vi "Drop Message Core.vi"(11 "Process Job Msg in":refnum<class "Process Job Msg.lvclass">) -> ()   [LabVIEW 2023, in "Worker.lvlib" / "Process Job Msg.lvclass"]
doc: "(<B>Filename</B>: Actor Framework.lvlib:Message.lvclass:Drop Message Core.vi)\n\nDefines what a message does if it is in the message queue when the queue is released. At this point, the actor has shut down, so it will never process the message.\n\nBy default, this method does nothing. A child class may override it to define behavior. National Instruments provides the Reply Msg class to override this method. This class releases its internal queue, which causes any caller of the Send Message and Wait For Response method to stop waiting and return an error."
uses:
  Process Job Msg.lvclass
  <vilib>/ActorFramework/Message/Message.lvclass
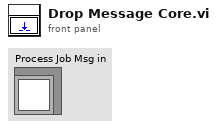
[diagram p1: front panel]
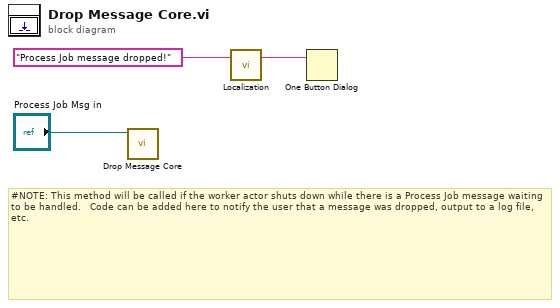
[diagram p0: block diagram]
diagram:
  # "#NOTE: This method will be called if the worker actor shuts down while there is a Process Job message waiting to be handled.   Code can be added here to notify the user that a message was dropped, output to a log file, etc."
  n1 = call-parent "Drop Message Core.vi"("Message in"="Process Job Msg in") -> ()  [unwired: 11 in]
  n2 = call "Localization.vi"("untranslated"="Process Job message dropped!" ("string")) -> ("translated"=w1:string)  [unwired: 2 in]
  n3 = One Button Dialog(message=w1) -> ()  [unwired: 1 in, 1 out]
